vi "Write Robodolf Controller State message.vi"(8 "error in (no error)":errorcluster, 10 "Controller":T1, 11 "Controller State in":refnum<class "Controller State.lvclass">) -> (0 "error out":errorcluster, 3 "Controller State out":refnum<class "Controller State.lvclass">)   [LabVIEW 2015, in "RDS Child Messages.lvlib" / "Controller State.lvclass"]
uses:
  Controller State.lvclass
  Actors/RDS Controller Actor/RDS Controller Actor/Controller.ctl
  Controller State.lvclass/Controller State.ctl
  Actors/RDS Controller Actor/RDS Controller Actor/RDS Controller Actor.lvlib
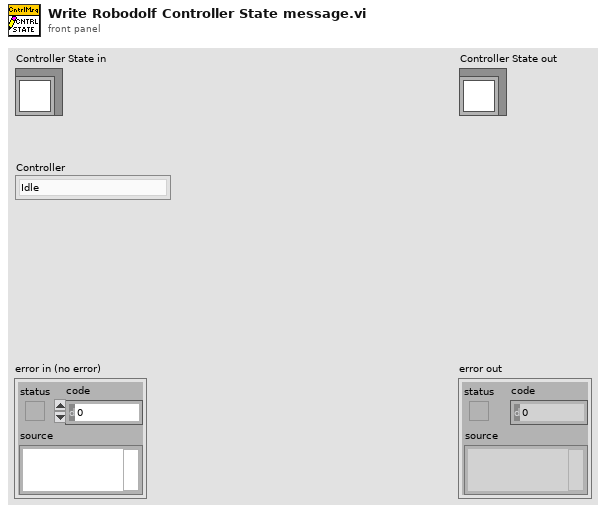
[diagram p1: front panel]
types:
  T1 = typedef "RDS Controller Actor.lvlib/Controller.ctl" = enum16{"Idle", "Local Remote Control", "Shore Remote Control", "Mission Control"}
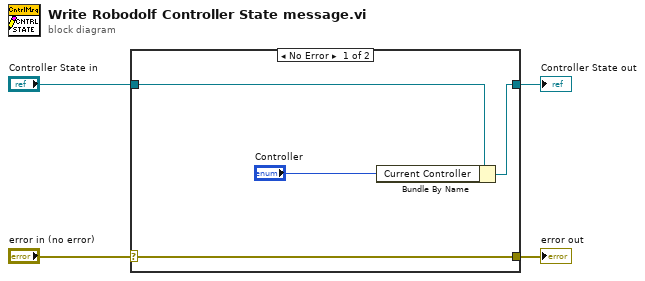
[diagram p0: block diagram]
diagram:
  n1 = case shown="No Error" "error in (no error)" {
    selector: "error in (no error)" -> [w8 w9]
    tunnel: [w8 w9] -> w3
    tunnel: [w6 w10] -> w1
    tunnel: "Controller State in" -> [w7 w10]
    frame No Error {
      n2 = Bundle By Name(cluster=w7, "Current Controller"="Controller") -> (w6:refnum<class "Controller State.lvclass">)
    }
    frame Error {
    }
  }
  "error out" <- w3
  "Controller State out" <- w1
